vi "Read Pulsed Current.vi"(0 "VISA resource name":refnum<visa-resource-name>, 1 "Pulse Off Time (0.4 S)":dbl=0.4, 2 "Pulse On Time (0.02 S)":dbl=0.02, 5 "Source Measure Unit Channel (0: Channel A)":i32(ring) items=["Channel A", "Channel B"], 7 "Bias Level (0 A)":dbl, 9 "Pulse Level (1 V)":dbl=1.0, 11 "error in (no error)":errorcluster, 12 "Sweep Points (10)":i32=10) -> (4 "VISA resource name out":refnum<visa-resource-name>, 6 "Current (A)":dbl[](array[numeric]), 15 "error out":errorcluster)   [LabVIEW 2020, in "Keithley 2600 Series.lvlib"]
doc: "Performs a voltage pulse with a current measurement cycles."
uses:
  <instrlib>/Keithley 2600 Series/Keithley 2600 Series.lvlib
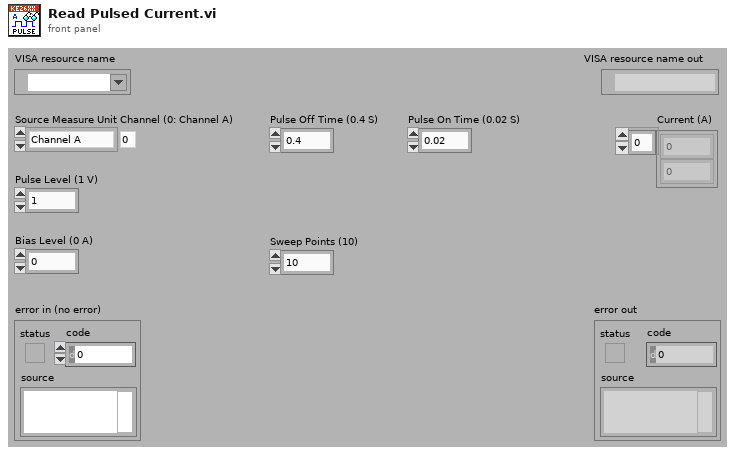
[diagram p1: front panel]
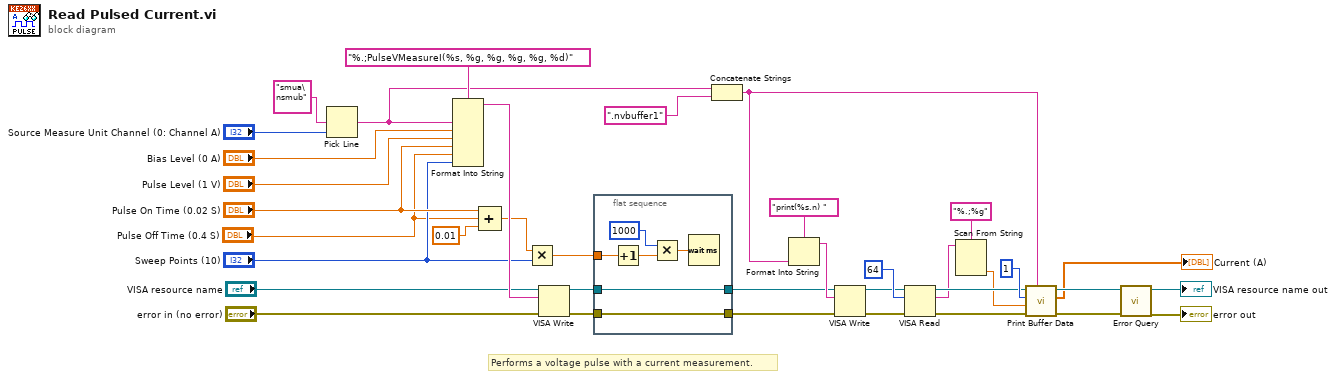
[diagram p0: block diagram]
diagram:
  # "Performs a voltage pulse with a current measurement."
  n1 = Pick Line(multi-line string="smua\nsmub", line index="Source Measure Unit Channel (0: Channel A)") -> (output string=w9:string)  [unwired: 1 in]
  n2 = Format Into String(format string="%.;PulseVMeasureI(%s, %g, %g, %g, %g, %d)", w9, "Bias Level (0 A)", "Pulse Level (1 V)", "Pulse On Time (0.02 S)", "Pulse Off Time (0.4 S)", "Sweep Points (10)") -> (resulting string=w34:string)  [unwired: 2 in, 1 out]
  n3 = Compound Arithmetic op=ADD("Pulse On Time (0.02 S)", "Pulse Off Time (0.4 S)", 0.01 ("value")) -> (w23:dbl)
  n4 = Multiply(x=w23, y="Sweep Points (10)") -> (x*y=w21:dbl)
  n5 = VISA Write(VISA resource name="VISA resource name", write buffer=w34, error in (no error)="error in (no error)") -> (VISA resource name out=w27:refnum<visa-resource-name>, error out=w26:errorcluster)  [unwired: 1 out]
  n6 = flat-sequence {
    tunnel: w27 -> [w43]
    tunnel: w26 -> [w42]
    tunnel: [w43] -> w7
    tunnel: [w42] -> w6
    tunnel: w21 -> [w39]
    frame #0 {
      n7 = Increment(x=w39) -> (x+1=w38:dbl)
      n8 = Multiply(x=1000, y=w38) -> (x*y=w40:dbl)
      n9 = Wait (ms)(milliseconds to wait=w40) -> ()  [unwired: 1 out]
    }
  }
  n10 = Concatenate Strings(w9, ".nvbuffer1" ("string")) -> (w3:string)
  n11 = Format Into String(format string="print(%s.n) ", w3) -> (resulting string=w10:string)  [unwired: 2 in, 1 out]
  n12 = VISA Write(VISA resource name=w7, write buffer=w10, error in (no error)=w6) -> (VISA resource name out=w13:refnum<visa-resource-name>, error out=w12:errorcluster)  [unwired: 1 out]
  n13 = VISA Read(VISA resource name=w13, byte count=u32 64, error in (no error)=w12) -> (VISA resource name out=w18:refnum<visa-resource-name>, read buffer=w16:string, error out=w17:errorcluster)  [unwired: 1 out]
  n14 = Scan From String(format string="%.;%g", input string=w16) -> (output 1=w15:dbl)  [unwired: 3 in, 3 out]
  n15 = call <instrlib>:"Print Buffer Data.vi"("Reading Buffer (smua.nvbuffer1)"=w3, "error in (no error)"=w17, "End Index (1)"=w15, "Start Index (1)"=1 ("Start Index (0)"), "VISA resource name"=w18) -> ("error out"=w4:errorcluster, "Buffer Data"=→"Current (A)":dbl[], "VISA resource name out"=w5:refnum<visa-resource-name>)  [unwired: 4 in]
  n16 = call <instrlib>:"Error Query.vi"("error in (no error)"=w4, "VISA resource name"=w5) -> ("error out"=→"error out":errorcluster, "VISA resource name out"=→"VISA resource name out":refnum<visa-resource-name>)  [unwired: 6 in, 2 out]
